vi "Yokogawa WT300 Series Measure Harmonics.vi"() -> ()   [LabVIEW 2019]
doc: "This example shows how to measure the harmonic measurement numeric list data.\n\n<b>Note:</b>\nThis setting valid on models with the harmonic measurement (/G5) option."
uses:
  Public/Data/Read Measurement (Harmonics).vi
  Yokogawa WT300 Series.lvlib
panel:
  in  "Function (0: None)":i32(ring) items=["None", "U", "I", "P", "Phi U", "Phi I", "UHDF", "IHDF", "PHDF"]
  in  "Element (1:1)":i32(ring)=1 items=["1"=1, "2"=2, "3"=3]
  in  "Max Order (0: All)":i32 min=0 max=50
  out "Measurement":dbl[](array[numeric])
  out "Function":string
  in  "Item (1)":i32=1 min=1 max=32 step=1
  in  "Timeout (10000 ms)":i32=10000 min=1
  in  "VISA resource name":refnum<visa-resource-name>
  # "(c) 2013 Yokogawa Meters & Instruments Corporation.  All rights reserved."
  # "WT300 SERIES POWER ANALYZER"
  # "Total        DC            1             2              3             4"
  # "ms"
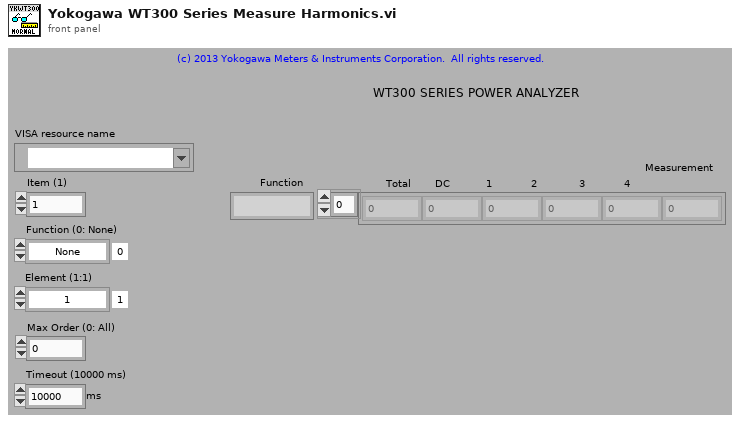
[diagram p1: front panel]
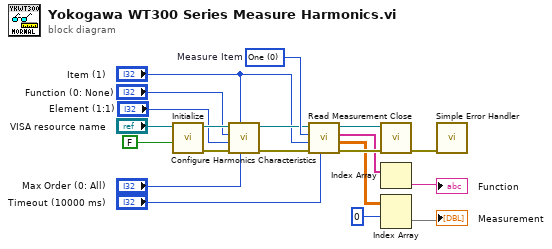
[diagram p0: block diagram]
diagram:
  w15 = 0 items=["One", "Plural"]  # Measure Item
  n1 = call "Initialize.vi"("Reset (True)"=FALSE ("Reset? (True)"), "VISA resource name"="VISA resource name") -> ("error out"=w8:errorcluster, "VISA resource name out"=w7:refnum<visa-resource-name>)  [unwired: 7 in, 1 out]
  n2 = call "Configure Harmonics Characteristics.vi"("Max Order (0: All)"="Max Order (0: All)", "Item (1)"="Item (1)", "error in (no error)"=w8, "Element (1:1)"="Element (1:1)", "Function (0: None)"="Function (0: None)", "VISA resource name"=w7) -> ("error out"=w3:errorcluster, "VISA resource name out"=w6:refnum<visa-resource-name>)  [unwired: 4 in]
  n3 = call-poly "Read Measurement.vi"("Timeout (10000 ms)"="Timeout (10000 ms)", "error in (no error)"=w3, "Number of Item (15)"="Item (1)", "Measure Item (1: Plural)"=w15, "VISA resource name"=w6) -> ("error out"=w17:errorcluster, "Measurement"=w14:dbl[][], "Function"=w12:string[], "VISA resource name out"=w18:refnum<visa-resource-name>)  [unwired: 3 in]
  n4 = call "Close.vi"("error in (no error)"=w17, "VISA resource name"=w18) -> ("error out"=w20:errorcluster)  [unwired: 9 in]
  n5 = Index Array(array=w12) -> (element=→"Function":string)  [unwired: 1 in]
  n6 = Index Array(array=w14, index (row)=0 ("指標 （行）")) -> (element=→"Measurement":dbl[])  [unwired: 1 in]
  n7 = call <vilib>:"Simple Error Handler.vi"("error in (no error)"=w20) -> ()  [unwired: 4 in, 5 out]
